vi "PART_II.vi"() -> ()   [LabVIEW 2019]
panel:
  out "ForLoop \nOutput":dbl[][](array[numeric])
  out "Output Array":dbl[](array[numeric])
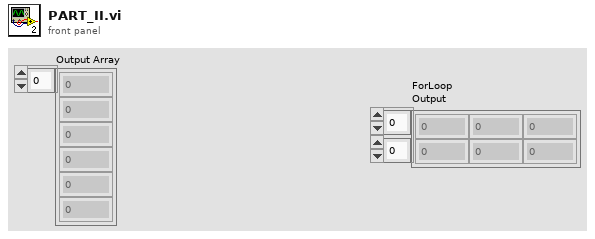
[diagram p1: front panel]
types:
  T1 = typedef "NI_Matrix.lvlib/RealMatrix.ctl" = dbl[][]
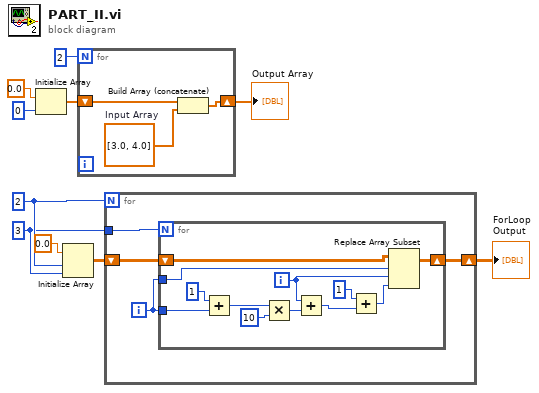
[diagram p0: block diagram]
diagram:
  w3 = 3
  w4 = 2
  n1 = Initialize Array(0.0 ("element"), 0 ("dimension size")) -> (w7:dbl[])
  n2 = Initialize Array(0.0 ("element"), w4, w3) -> (w2:dbl[][])
  n3 = for {
    N: 2 -> [_]
    shift-right: [w12] -> w6
    shift-left: w7 -> [w11]
    w13 = dbl[] [3.0, 4.0]  # Input Array
    n4 = Build Array (concatenate)(w11, w13) -> (w12:dbl[])
  }
  "Output Array" <- w6
  n5 = for {
    N: w4 -> [_]
    tunnel: w3 -> [w17]
    shift-right: [w15] -> w1
    shift-left: w2 -> [w16]
    i -> [w14]
    n6 = for {
      N: w17 -> [_]
      shift-right: [w28] -> w15
      shift-left: w16 -> [w29]
      tunnel: w14 -> [w27]
      tunnel: w14 -> [w25]
      i -> [w21]
      n7 = Add(x=1, y=w25) -> (x+y=w24:i32)
      n8 = Multiply(x=w24, y=10) -> (x*y=w22:i32)
      n9 = Add(x=w21, y=w22) -> (x+y=w20:i32)
      n10 = Add(x=1, y=w20) -> (x+y=w18:i32)
      n11 = Replace Array Subset(array=w29, new element=w18, index (row)=w27, index (col)=w21) -> (w28:T1)
    }
  }
  "ForLoop \nOutput" <- w1
